vi "Write header ccd configuration.vi"(8 "error in (no error)":errorcluster, 11 "CCDCamera in":refnum<class "CCDCamera.lvclass">) -> (0 "error out":errorcluster, 3 "CCDCamera out":refnum<class "CCDCamera.lvclass">)   [LabVIEW 2018, in "CCDCamera.lvclass"]
uses:
  CCDCamera.lvclass
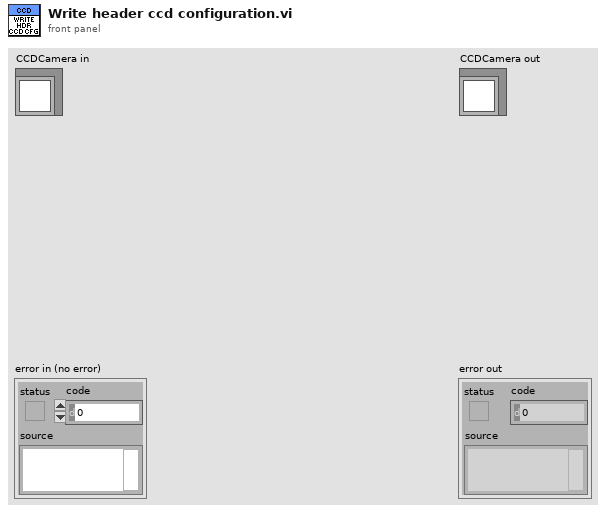
[diagram p1: front panel]
types:
  T1 = cluster{"PREAMP":u16, "READOUT_RATE":u16, "EM_GAIN":u16, "VERTICAL_SHIFT_SPEED":u16, "READ_MODE":u16, "FRAME_TRANSFER":bool, "VERTICAL_CLOCK_VOLTAGE":u16, "ACQUISITION_MODE":u16, "AD_CHANNEL":u16, "EM_MODE":u16, "SHUTTER_TTL":u16, "SHUTTER_OPENING_TIME":u16, "SHUTTER_CLOSING_TIME":u16, "SHUTTER_MODE":u16, "TRIGGER_MODE":u16, "VBIN":u16, "INITIAL_LINE":u16, "INITIAL_COLUMN":u16, "FINAL_LINE":u16, "FINAL_COLUMN":u16, "HBIN":u16}
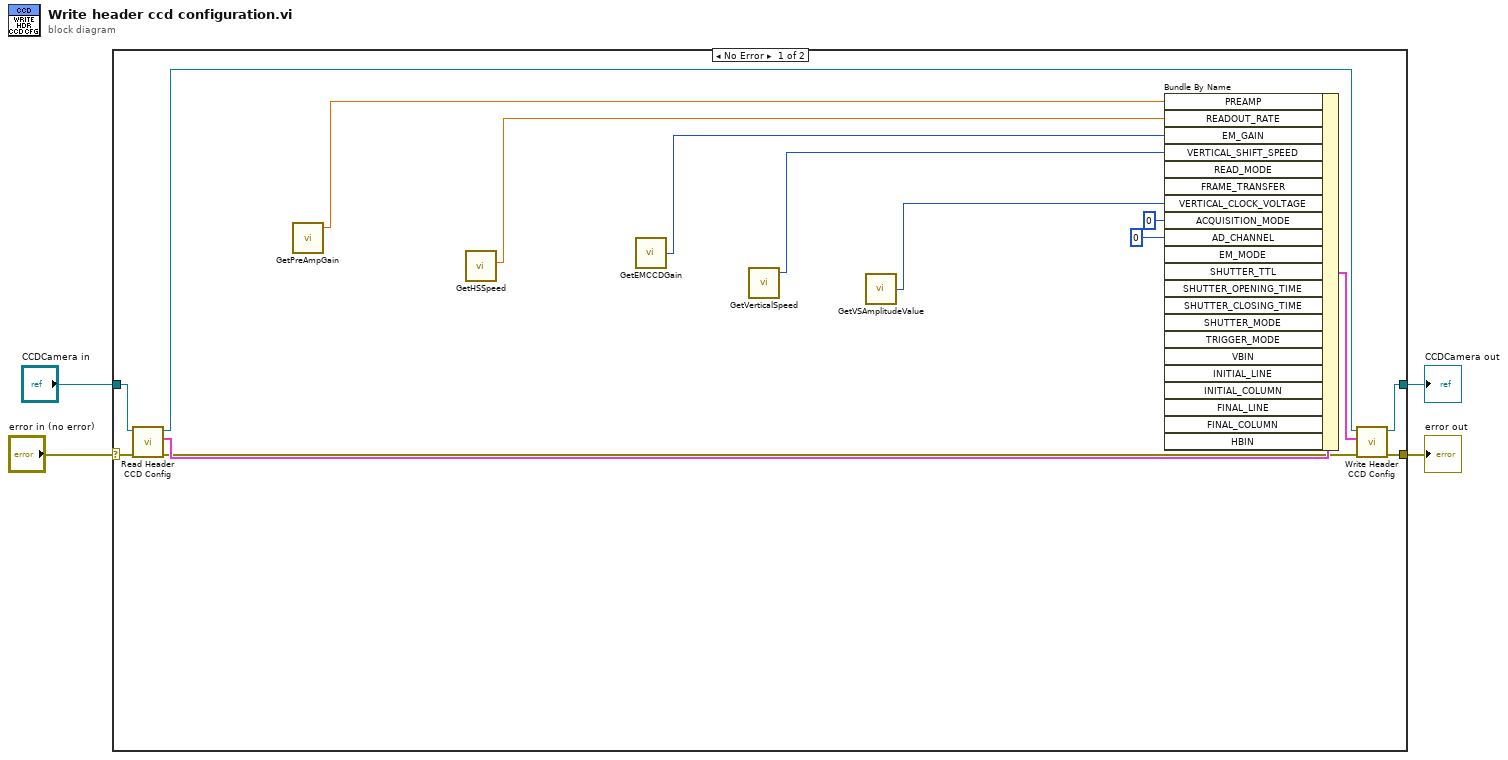
[diagram p0: block diagram]
diagram:
  n1 = case shown="No Error" "error in (no error)" {
    selector: "error in (no error)" -> [w15 w20]
    tunnel: "CCDCamera in" -> [w16 w21]
    tunnel: [w17 w21] -> w2
    tunnel: [w13 w20] -> w1
    frame No Error {
      n2 = call-dynamic "Read Header CCD Config.vi"("error in (no error)"=w15, "Simulated_CCD_Camera in"=w16) -> ("error out"=w14:errorcluster, "Header CCD Config"=w19:T1, "Simulated_CCD_Camera out"=w18:refnum<class "CCDCamera.lvclass">)  [unwired: 7 in]
      n3 = call <userlib>:"GetPreAmpGain.vi"() -> ("gain"=w11:sgl)  [unwired: 3 in, 2 out]
      n4 = call <userlib>:"GetHSSpeed.vi"() -> ("speed"=w10:sgl)  [unwired: 5 in, 2 out]
      n5 = call <userlib>:"GetEMCCDGain.vi"() -> ("gain"=w9:u32)  [unwired: 3 in, 2 out]
      n6 = call <userlib>:"GetVerticalSpeed.vi"() -> ("speed"=w8:i32)  [unwired: 2 in, 2 out]
      n7 = call <userlib>:"GetVSAmplitudeValue.vi"() -> ("value"=w7:i32)  [unwired: 2 in, 2 out]
      n8 = Bundle By Name(cluster=w19, "PREAMP"=w11, "READOUT_RATE"=w10, "EM_GAIN"=w9, "VERTICAL_SHIFT_SPEED"=w8, "VERTICAL_CLOCK_VOLTAGE"=w7, "ACQUISITION_MODE"=u16 0, "AD_CHANNEL"=u16 0) -> (w12:T1)  [unwired: 14 in]
      n9 = call-dynamic "Write Header CCD Config.vi"("error in (no error)"=w14, "Header CCD Config"=w12, "Simulated_CCD_Camera in"=w18) -> ("error out"=w13:errorcluster, "Simulated_CCD_Camera out"=w17:refnum<class "CCDCamera.lvclass">)  [unwired: 7 in]
    }
    frame Error {
    }
  }
  "error out" <- w1
  "CCDCamera out" <- w2
